vi "type_05_uint8_two_segments.vi"() -> ()   [LabVIEW 2010]
panel:
  out "error out":errorcluster
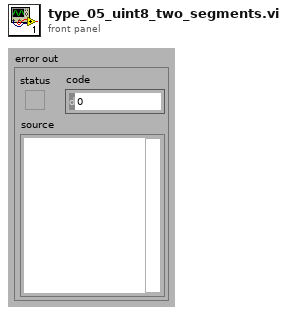
[diagram p1: front panel]
types:
  T1 = enum16{"open", "open or create", "create or replace", "create", "open (read-only)"}
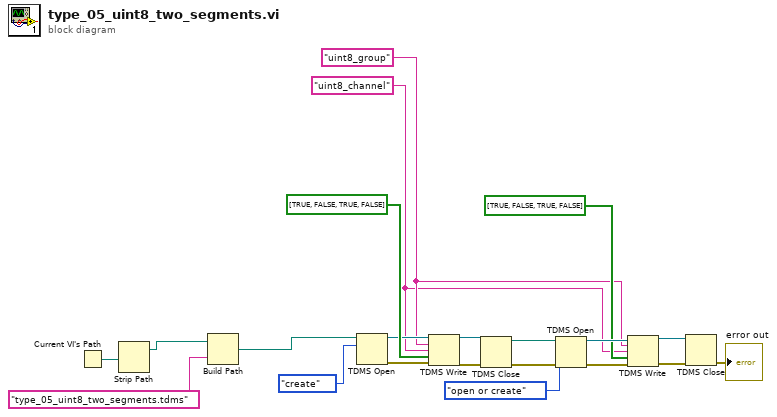
[diagram p0: block diagram]
diagram:
  w1 = "uint8_channel" ("channel name(s) in (Untitled)")
  w2 = "uint8_group" ("group name in (Untitled)")
  n1 = Current VI's Path() -> (path=w20:path)
  n2 = Strip Path(path=w20) -> (stripped path=w19:path)  [unwired: 1 out]
  n3 = Build Path(base path=w19, name or relative path="type_05_uint8_two_segments.tdms") -> (appended path=w17:path)
  n4 = TDMS Open(10:T1."create" ("operation (0:open)"), 11:w17) -> (0:w4:errorcluster, 3:w3:refnum<k34>)  [unwired: 4 in]
  n5 = TDMS Write(0:w3, 5:w2, 7:w1, 9:bool[] [TRUE, FALSE, TRUE, FALSE], 11:w4) -> (4:w5:refnum<k34>, 15:w6:errorcluster)  [unwired: 1 in, 2 out]
  n6 = TDMS Close(8:w6, 11:w5) -> (0:w14:errorcluster, 3:w16:path)
  n7 = TDMS Open(8:w14, 10:T1."open or create" ("operation (0:open)"), 11:w16) -> (0:w13:errorcluster, 3:w12:refnum<k34>)  [unwired: 3 in]
  n8 = TDMS Write(0:w12, 5:w2, 7:w1, 9:bool[] [TRUE, FALSE, TRUE, FALSE], 11:w13) -> (4:w10:refnum<k34>, 15:w11:errorcluster)  [unwired: 1 in, 2 out]
  n9 = TDMS Close(8:w11, 11:w10) -> (0:→"error out":errorcluster)  [unwired: 1 out]
